vi "RunTestItems.vi"(6 "seconds since 1Jan1904":timestamp, 7 "Multicolumn Listbox":refnum<vi>, 8 "error in (no error)":errorcluster, 9 "Item in":string[][](array[string]), 10 "ItemNames":string[][](array[string]), 11 "steps":i32) -> (0 "error out":errorcluster, 1 "Items out":string[][](array[string]), 2 "Horizontal Graduated Bar":u8(slide) max=28 scale=-1.0..7.0, 3 "Result":string, 4 "Result":bool[](array[boolean]), 5 "Multicolumn Listbox 2":refnum<vi>)   [LabVIEW 2013]
uses:
  <vilib>/Utility/miscctls.llb/LVRowAndColumnTypeDef.ctl
  SubVi/Global constant.vi
panel:
  out "Test Time":string
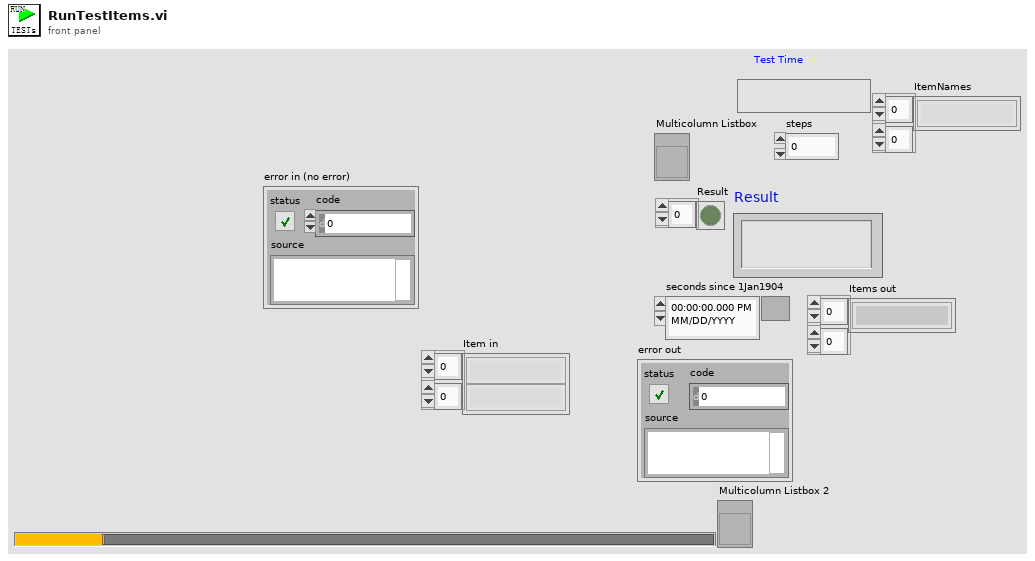
[diagram p1: front panel]
types:
  T1 = cluster{"step name 1":string, "updata 2":string, "limitdata 3":string, "load vi name 4":string, "parameter 5":string}
  T2 = cluster{"concatenated string":string, "Result":bool}
  T3 = typedef "LVRowAndColumnTypeDef.ctl" = cluster{"Row":i32, "Column":i32}
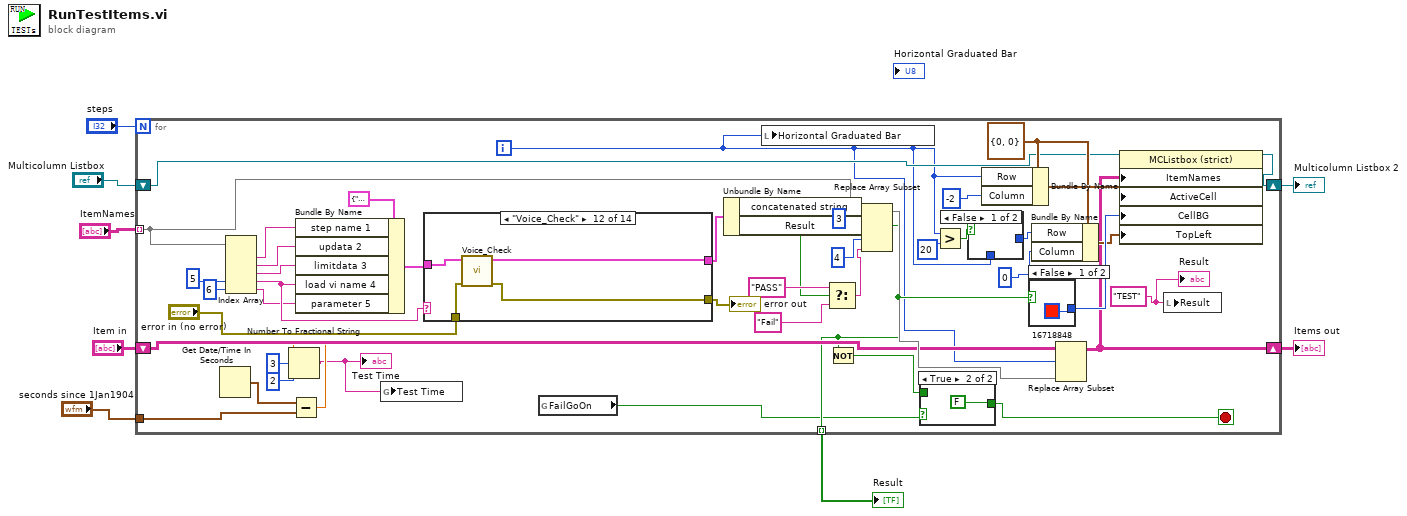
[diagram p0: block diagram]
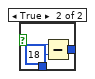
[diagram p3: hidden frame]
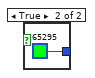
[diagram p4: hidden frame]
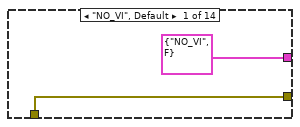
[diagram p5: hidden frame]
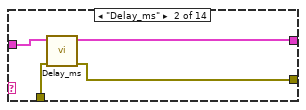
[diagram p6: hidden frame]
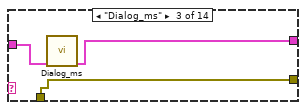
[diagram p7: hidden frame]
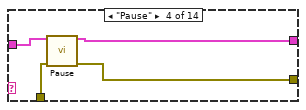
[diagram p8: hidden frame]
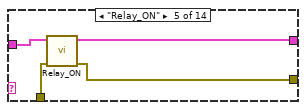
[diagram p9: hidden frame]
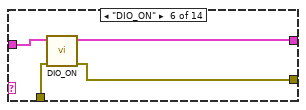
[diagram p10: hidden frame]
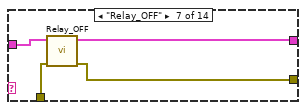
[diagram p11: hidden frame]
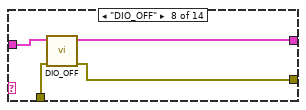
[diagram p12: hidden frame]
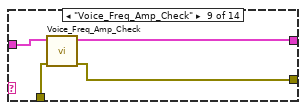
[diagram p13: hidden frame]
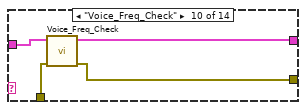
[diagram p14: hidden frame]
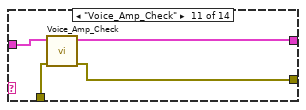
[diagram p15: hidden frame]
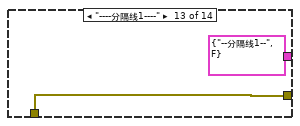
[diagram p16: hidden frame]
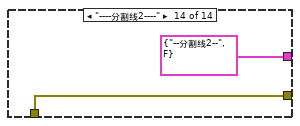
[diagram p17: hidden frame]
diagram:
  n1 = for {
    N: "steps" -> [_]
    tunnel: "ItemNames" -> [w30] mode=indexing
    shift-right: [w28] -> w3
    shift-left: "Item in" -> [w29]
    shift-right: [w27] -> w1
    shift-left: "Multicolumn Listbox" -> [w31]
    tunnel: [w24] -> w2 mode=indexing
    tunnel: "seconds since 1Jan1904" -> [w22]
    i -> [w23]
    stop <- w26 stop-if-true
    w13 = "TEST"
    w38 = T3 {"Row"=0, "Column"=0} ("Active Cell:Active Cell")
    n2 = Get Date/Time In Seconds() -> (seconds since 1Jan1904=w21:timestamp)
    n3 = Index Array(array=w30, index #4=5 ("index"), index #5=6 ("index")) -> (element #1=w52:string, element #2=w51:string, element #3=w50:string, element #4=w17:string, element #5=w16:string)  [unwired: 3 in]
    n4 = Subtract(x=w21, y=w22) -> (x-y=w20:dbl)
    n5 = Number To Fractional String(number=w20, width (-)=i16 3, precision (6)=i16 2) -> (F-format string=w9:string)  [unwired: 1 in]
    "Test Time" <- w9
    n6 = Bundle By Name(cluster=T1 {"step name 1"="", "updata 2"="", "limitdata 3"="", "load vi name 4"="", "parameter 5"=""} ("IN"), "step name 1"=w52, "updata 2"=w51, "limitdata 3"=w50, "load vi name 4"=w17, "parameter 5"=w16) -> (w49:T1)
    n7 = global write "Global constant.vi" "Test Time"(w9) -> ()
    n8 = case shown="\"Voice_Check\"" w17 {
      tunnel: w49 -> [_ w66 w69 w73 w77 w81 w85 w89 w93 w97 w101 w105 _ _]
      tunnel: [w62 w65 w67 w70 w76 w80 w84 w88 w92 w96 w100 w104 w107 w109] -> w11
      tunnel: [T2 {"concatenated string"="NO_VI", "Result"=FALSE} ("Cluster") w64 w68 w72 w75 w79 w83 w87 w91 w95 w99 w103 T2 {"concatenated string"="--分隔线1--", "Result"=FALSE} ("Cluster") T2 {"concatenated string"="--分割线2--", "Result"=FALSE} ("Cluster")] -> w32
      tunnel: "error in (no error)" -> [w62 w63 w67 w71 w74 w78 w82 w86 w90 w94 w98 w102 w107 w109]
      frame "NO_VI", Default {
      }
      frame "Delay_ms" {
        n9 = call "Delay_ms.vi"("error in (no error)"=w63, "IN"=w66) -> ("error out"=w65:errorcluster, "Cluster"=w64:T2)  [unwired: 8 in]
      }
      frame "Dialog_ms" {
        n10 = call "Dialog_ms.vi"("IN"=w69) -> ("Cluster"=w68:T2)  [unwired: 8 in, 2 out]
      }
      frame "Pause" {
        n11 = call "Pause.vi"("IN"=w73, "error in (no error)"=w71) -> ("Cluster"=w72:T2, "error out"=w70:errorcluster)  [unwired: 12 in]
      }
      frame "Relay_ON" {
        n12 = call "Relay_ON.vi"("error in (no error)"=w74, "IN"=w77) -> ("error out"=w76:errorcluster, "Cluster"=w75:T2)  [unwired: 8 in]
      }
      frame "DIO_ON" {
        n13 = call "DIO_ON.vi"("error in (no error)"=w78, "IN"=w81) -> ("error out"=w80:errorcluster, "Cluster"=w79:T2)  [unwired: 8 in]
      }
      frame "Relay_OFF" {
        n14 = call "Relay_OFF.vi"("error in (no error)"=w82, "IN"=w85) -> ("error out"=w84:errorcluster, "Cluster"=w83:T2)  [unwired: 8 in]
      }
      frame "DIO_OFF" {
        n15 = call "DIO_OFF.vi"("error in (no error)"=w86, "IN"=w89) -> ("error out"=w88:errorcluster, "Cluster"=w87:T2)  [unwired: 8 in]
      }
      frame "Voice_Freq_Amp_Check" {
        n16 = call "Voice_Freq_Amp_Check.vi"("error in (no error)"=w90, "IN"=w93) -> ("error out"=w92:errorcluster, "Cluster"=w91:T2)  [unwired: 8 in]
      }
      frame "Voice_Freq_Check" {
        n17 = call "Voice_Freq_Check.vi"("error in (no error)"=w94, "IN"=w97) -> ("error out"=w96:errorcluster, "Cluster"=w95:T2)  [unwired: 8 in]
      }
      frame "Voice_Amp_Check" {
        n18 = call "Voice_Amp_Check.vi"("error in (no error)"=w98, "IN"=w101) -> ("error out"=w100:errorcluster, "Cluster"=w99:T2)  [unwired: 8 in]
      }
      frame "Voice_Check" {
        n19 = call "Voice_Check.vi"("error in (no error)"=w102, "IN"=w105) -> ("error out"=w104:errorcluster, "Cluster"=w103:T2)  [unwired: 8 in]
      }
      frame "----分隔线1----" {
      }
      frame "----分割线2----" {
      }
    }
    "error out" <- w11
    n20 = global read "Global constant.vi" "FailGoOn"() -> (w10:bool)
    n21 = Unbundle By Name(w32) -> ("concatenated string"=w47:string, "Result"=w24:bool)
    n22 = local write "Horizontal Graduated Bar"(w23) -> ()
    n23 = Select(t="PASS", s=w24, f="Fail") -> (s? t:f=w43:string)
    n24 = Not(x=w24) -> (.not. x?=w25:bool)
    n25 = Replace Array Subset(array=w30, new element #1=w47, index #1=3 ("index"), new element #2=w43, index #2=4 ("index")) -> (w42:string[])
    n26 = case shown="True" w10 {
      tunnel: [w54 FALSE] -> w26
      tunnel: w25 -> [w54 _]
      frame False {
      }
      frame True {
      }
    }
    n27 = Greater?(x=w23, y=20) -> (0:w34:bool)
    n28 = case shown="False" w34 {
      tunnel: w23 -> [_ w58]
      tunnel: [_ w56] -> w33
      frame False {
      }
      frame True {
        n29 = Subtract(x=w58, y=18) -> (x-y=w56:i32)
      }
    }
    n30 = Bundle By Name(cluster=w38, "Row"=w23, "Column"=-2) -> (w39:T3)
    n31 = case shown="False" w24 {
      tunnel: [u32 16718848 u32 65295] -> w41
      frame False {
      }
      frame True {
      }
    }
    n32 = Bundle By Name(cluster=w38, "Row"=w33, "Column"=0) -> (w37:T3)
    n33 = Replace Array Subset(array=w29, new element=w42, index (row)=w23) -> (w28:string[][])  [unwired: 1 in]
    n34 = property class="MCListbox (strict)"(reference=w31, "ItemNames"=w28, "ActiveCell"=w39, "CellBG"=w41, "TopLeft"=w37) -> (reference out=w27:refnum<vi>)  [unwired: 1 in, 1 out]
    n35 = local write "Result"(w13) -> ()
    "Result" <- w13
  }
  "Items out" <- w3
  "Result" <- w2
  "Multicolumn Listbox 2" <- w1
